vi "DAQmx Create Channel (TEDS-AI-Temperature-RTD).vi"(0 "task in":refnum<k21>, 1 "maximum value":dbl=100.0 format="%0.2f", 2 "minimum value":dbl format="%0.2f", 3 "resistance configuration":i32(ring)=2 items=["2-Wire"=2, "3-Wire"=3, "4-Wire"=4], 5 "physical channels":tag, 7 "name to assign":string, 9 "units":i32(ring)=10143 items=["Deg C"=10143, "Deg F"=10144, "Kelvins"=10325, "Deg R"=10145, "From Custom Scale"=10065], 10 "current excitation value":dbl=0.0025 format="%0.5f", 11 "error in":errorcluster, 13 "current excitation source":i32(ring)=10167 items=["Internal"=10200, "External"=10167, "None"=10230]) -> (4 "task out":refnum<k21>, 15 "error out":errorcluster)   [LabVIEW 2018]
doc: "Creates channel(s) that use an RTD to measure temperature. You must configure the physical channel(s) with TEDS information to use this VI."
uses:
  nilvaiu.dll
panel:
  # "input limits"
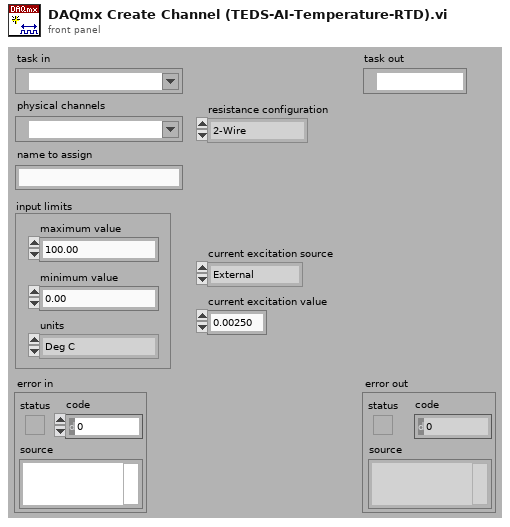
[diagram p1: front panel]
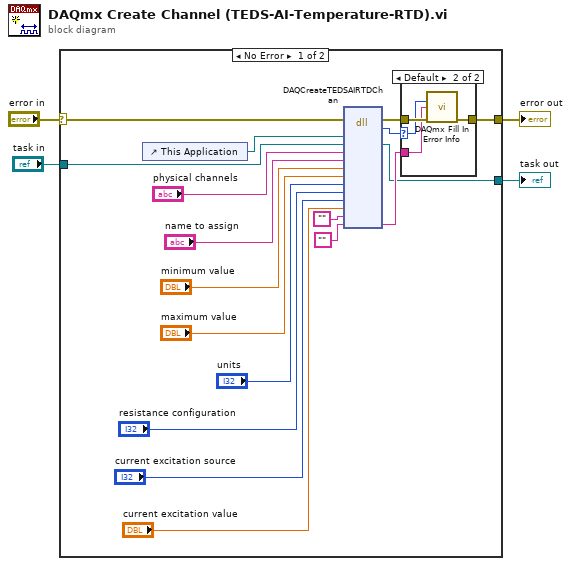
[diagram p0: block diagram]
diagram:
  n1 = case shown="No Error" "error in" {
    selector: "error in" -> [w7 w28]
    tunnel: "task in" -> [w10 w29]
    tunnel: [w9 w29] -> w3
    tunnel: [w8 w28] -> w2
    frame No Error {
      n2 = control-ref of="This Application"() -> (w18:refnum<vi>)
      n3 = dll-call lib="nilvaiu.*" fn="DAQCreateTEDSAIRTDChan"(error in=w7, "lvAppRef"=w18, "refObjPtr"=w10, "physicalChannelName"="physical channels", "channelNameIn"="name to assign", "minVal"="minimum value", "maxVal"="maximum value", "units"="units", "resistanceConfig"="resistance configuration", "currentExcitSource"="current excitation source", "currentExcitVal"="current excitation value", "channelNamesOut"="", "extenededErrorInfo"="") -> (error out=w22:errorcluster, "return type"=w21:i32, "refObjPtr"=w9:refnum<k21>, "extenededErrorInfo"=w17:string)  [unwired: 12 in, 1 out]
      n4 = case shown="Default" w21 {
        selector: w21 -> [_ w25]
        tunnel: w22 -> [w23 w27]
        tunnel: [w23 w26] -> w8
        tunnel: w17 -> [_ w24]
        frame 0 {
        }
        frame Default {
          n5 = call "DAQmx Fill In Error Info.vi"("status code"=w25, "extended error info"=w24, "error in"=w27) -> ("error out"=w26:errorcluster)  [unwired: 1 in, 11 out]
        }
      }
    }
    frame Error {
    }
  }
  "task out" <- w3
  "error out" <- w2
